vi "Write_LS_Data.vi"(1 "In":T1={"Time"=[], "LI1CH1"=[], "LI1CH2"=[], "LI2CH1"=[], "LI2CH2"=[], "LI3CH1"=[], "LI3CH2"=[], "Field"=[], "N_Level"=[], "H_Level"=[], "Heat_370"=[], "Sorb_Heat"=[], "Still_Heat"=[], "Capacity"=[], "Loss"=[], "Magnet_Temperature"=[], "Lam_Pressure"=[], "Lam_NValve"=[], "370-T1"=[], "370-T2"=[], "370-T3"=[], "370-T4"=[], "370-T5"=[], "370-R1"=[], "370-R2"=[], "370-R3"=[], "370-R4"=[], "370-R5"=[], "372-T1"=[], "372-T2"=[], "372-T3"=[], "372-T4"=[], "372-T5"=[], "372-T6"=[], "372-R1"=[], "372-R2"=[], "372-R3"=[], "372-R4"=[], "372-R5"=[], "372-R6"=[], "Nada"=[nan], "K2440_Res"=[], "K2440_Current"=[], "VTI_Heater"=[], "VTI_NValve"=[], "LS340_Heater"=[], "K6221_Amplitude"=[], "K6221_Frequency"=[], "Cond_Pressure"=[], "Still_Pressure"=[], "FP_Out_Pressure"=[], "Dump_Pressure"=[], "V1"=[], "V2"=[], "V4"=[], "V5"=[], "V9"=[], "Forepump"=[], "Compressor"=[], "K6221_Offset"=[], "BoxTemp"=[], "By"=[], "Bz"=[], "Phi"=[], "heater-recond (%)"=[], "Dewar Pressure "=[], "JT-SP-Control"=[], "350 T1"=[], "350 T2"=[], "350 T3"=[], "350 T4"=[], "350 R1"=[], "350 R2"=[], "350 R3"=[], "350 R4"=[], "Angle"=[], "VTI CH1"=[], "VTI CH2"=[], "VTI CH3"=[], "ColdTrap"=[], "Mischer Pot"=[], "G1 (mbar)"=[], "G3 (mbar) "=[], "G4 (mbar)"=[], "IVC (mbar)"=[], "P2 (mbar) "=[], "Pot mischer (mbar)"=[], "AVS Control Channel (K)"=[], "AVS Control Channel (RES)"=[], "AVS  Channel 5 (RES) "=[], "LI3CH3"=[], "LI3CH4"=[], "LI1CH3"=[], "LI1CH4"=[], "LI2CH3"=[], "LI2CH4"=[], "Volt"=[], "Watt"=[], "Torque Angle"=[], "Dewar heater (W)"=[], "PSU Voltage"=[], "Turbopump"=[], "372-R7"=[], "372-T7"=[], "SIM921 Ch1"=[], " He3 Temp1"=[], " He3 Temp 2"=[], "LI4CH1"=[], "LI4CH2"=[], "372-T8"=[], "372-R8"=[]}) -> (0 "Out":T1={"Time"=[], "LI1CH1"=[], "LI1CH2"=[], "LI2CH1"=[], "LI2CH2"=[], "LI3CH1"=[], "LI3CH2"=[], "Field"=[], "N_Level"=[], "H_Level"=[], "Heat_370"=[], "Sorb_Heat"=[], "Still_Heat"=[], "Capacity"=[], "Loss"=[], "Magnet_Temperature"=[], "Lam_Pressure"=[], "Lam_NValve"=[], "370-T1"=[], "370-T2"=[], "370-T3"=[], "370-T4"=[], "370-T5"=[], "370-R1"=[], "370-R2"=[], "370-R3"=[], "370-R4"=[], "370-R5"=[], "372-T1"=[], "372-T2"=[], "372-T3"=[], "372-T4"=[], "372-T5"=[], "372-T6"=[], "372-R1"=[], "372-R2"=[], "372-R3"=[], "372-R4"=[], "372-R5"=[], "372-R6"=[], "Nada"=[nan], "K2440_Res"=[], "K2440_Current"=[], "VTI_Heater"=[], "VTI_NValve"=[], "LS340_Heater"=[], "K6221_Amplitude"=[], "K6221_Frequency"=[], "Cond_Pressure"=[], "Still_Pressure"=[], "FP_Out_Pressure"=[], "Dump_Pressure"=[], "V1"=[], "V2"=[], "V4"=[], "V5"=[], "V9"=[], "Forepump"=[], "Compressor"=[], "K6221_Offset"=[], "BoxTemp"=[], "By"=[], "Bz"=[], "Phi"=[], "heater-recond (%)"=[], "Dewar Pressure "=[], "JT-SP-Control"=[], "350 T1"=[], "350 T2"=[], "350 T3"=[], "350 T4"=[], "350 R1"=[], "350 R2"=[], "350 R3"=[], "350 R4"=[], "Angle"=[], "VTI CH1"=[], "VTI CH2"=[], "VTI CH3"=[], "ColdTrap"=[], "Mischer Pot"=[], "G1 (mbar)"=[], "G3 (mbar) "=[], "G4 (mbar)"=[], "IVC (mbar)"=[], "P2 (mbar) "=[], "Pot mischer (mbar)"=[], "AVS Control Channel (K)"=[], "AVS Control Channel (RES)"=[], "AVS  Channel 5 (RES) "=[], "LI3CH3"=[], "LI3CH4"=[], "LI1CH3"=[], "LI1CH4"=[], "LI2CH3"=[], "LI2CH4"=[], "Volt"=[], "Watt"=[], "Torque Angle"=[], "Dewar heater (W)"=[], "PSU Voltage"=[], "Turbopump"=[], "372-R7"=[], "372-T7"=[], "SIM921 Ch1"=[], " He3 Temp1"=[], " He3 Temp 2"=[], "LI4CH1"=[], "LI4CH2"=[], "372-T8"=[], "372-R8"=[]})   [LabVIEW 2019]
uses:
  Global/Global Variables/System Monitor Cluster.ctl
  Global/Global Variables/Data_Display_global.vi
  Instrument_Setup.vi
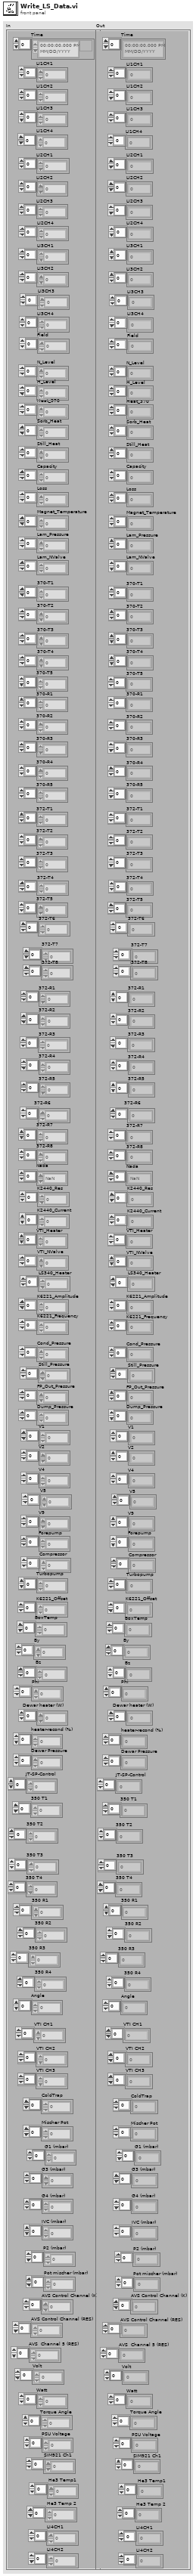
[diagram p1: front panel]
types:
  T1 = typedef "System Monitor Cluster.ctl" = cluster{"Time":timestamp[], "LI1CH1":dbl[], "LI1CH2":dbl[], "LI2CH1":dbl[], "LI2CH2":dbl[], "LI3CH1":dbl[], "LI3CH2":dbl[], "Field":dbl[], "N_Level":dbl[], "H_Level":dbl[], "Heat_370":dbl[], "Sorb_Heat":dbl[], "Still_Heat":dbl[], "Capacity":dbl[], "Loss":dbl[], "Magnet_Temperature":dbl[], "Lam_Pressure":dbl[], "Lam_NValve":dbl[], "370-T1":dbl[], "370-T2":dbl[], "370-T3":dbl[], "370-T4":dbl[], "370-T5":dbl[], "370-R1":dbl[], "370-R2":dbl[], "370-R3":dbl[], "370-R4":dbl[], "370-R5":dbl[], "372-T1":dbl[], "372-T2":dbl[], "372-T3":dbl[], "372-T4":dbl[], "372-T5":dbl[], "372-T6":dbl[], "372-R1":dbl[], "372-R2":dbl[], "372-R3":dbl[], "372-R4":dbl[], "372-R5":dbl[], "372-R6":dbl[], "Nada":dbl[], "K2440_Res":dbl[], "K2440_Current":dbl[], "VTI_Heater":dbl[], "VTI_NValve":dbl[], "LS340_Heater":dbl[], "K6221_Amplitude":dbl[], "K6221_Frequency":dbl[], "Cond_Pressure":dbl[], "Still_Pressure":dbl[], "FP_Out_Pressure":dbl[], "Dump_Pressure":dbl[], "V1":dbl[], "V2":dbl[], "V4":dbl[], "V5":dbl[], "V9":dbl[], "Forepump":dbl[], "Compressor":dbl[], "K6221_Offset":dbl[], "BoxTemp":dbl[], "By":dbl[], "Bz":dbl[], "Phi":dbl[], "heater-recond (%)":dbl[], "Dewar Pressure ":dbl[], "JT-SP-Control":dbl[], "350 T1":dbl[], "350 T2":dbl[], "350 T3":dbl[], "350 T4":dbl[], "350 R1":dbl[], "350 R2":dbl[], "350 R3":dbl[], "350 R4":dbl[], "Angle":dbl[], "VTI CH1":dbl[], "VTI CH2":dbl[], "VTI CH3":dbl[], "ColdTrap":dbl[], "Mischer Pot":dbl[], "G1 (mbar)":dbl[], "G3 (mbar) ":dbl[], "G4 (mbar)":dbl[], "IVC (mbar)":dbl[], "P2 (mbar) ":dbl[], "Pot mischer (mbar)":dbl[], "AVS Control Channel (K)":dbl[], "AVS Control Channel (RES)":dbl[], "AVS  Channel 5 (RES) ":dbl[], "LI3CH3":dbl[], "LI3CH4":dbl[], "LI1CH3":dbl[], "LI1CH4":dbl[], "LI2CH3":dbl[], "LI2CH4":dbl[], "Volt":dbl[], "Watt":dbl[], "Torque Angle":dbl[], "Dewar heater (W)":dbl[], "PSU Voltage":dbl[], "Turbopump":dbl[], "372-R7":dbl[], "372-T7":dbl[], "SIM921 Ch1":dbl[], " He3 Temp1":dbl[], " He3 Temp 2":dbl[], "LI4CH1":dbl[], "LI4CH2":dbl[], "372-T8":dbl[], "372-R8":dbl[]}
  T2 = typedef "LS372-Cluster.ctl" = cluster{"Activate Tsweep":bool, "Setpoint - Manual":dbl, "Rate (K/min)":dbl, "Update Lakeshores":bool, "Still Heater":bool, "Still Power (mW)":dbl, "Manual Heater":bool, "Manual Heater  (mW) ":dbl, "Heater Range":dbl, "P (Gain)":dbl, "I (Reset)":dbl, "D (Rate)":dbl, "Heater Power (mW)":dbl, "MC Thermometer":u16, "MC Temperature":dbl, "LS372-T1":dbl, "LS372 -T2":dbl, "LS372-R1 ":dbl, "LS372-R2":dbl, "LS372-T3":dbl, "LS372-T4":dbl, "LS372-R3 ":dbl, "LS372-R4 \n\n\n\n":dbl, "LS372-T5":dbl, "LS372-T6":dbl, "LS372-R5":dbl, "LS372-R6 ":dbl, "Still Power ist":dbl, "Set Temperatur Sweep main":bool, "Setpoint ist":dbl, "Disable Heater":bool}
  T3 = typedef "LS372_read_only-Cluster.ctl" = cluster{"LS372-T1":dbl, "LS372 -T2":dbl, "LS372-T4":dbl, "LS372-T5":dbl, "LS372-T6":dbl, "LS372-R1 ":dbl, "LS372-R2":dbl, "LS372-R3 ":dbl, "LS372-R4 \n\n\n\n":dbl, "LS372-R5":dbl, "LS372-R6 ":dbl, "LS372-T3":dbl, "Update Lakeshores":bool}
  T4 = typedef "LS370_only_readout_cluster.ctl" = cluster{"LS370 T1":dbl, "LS370 T2":dbl, "LS370 T3":dbl, "LS370 T4":dbl, "LS370 T5":dbl, "LS370 R1":dbl, "LS370 R2":dbl, "LS370 R3":dbl, "LS370 R4":dbl, "LS370 R5":dbl, "LS370 T6":dbl, "LS370 T7":dbl, "LS370 T8":dbl, "LS370 T9":dbl, "LS370 R6":dbl, "LS370 R7":dbl, "LS370 R8":dbl, "LS370 R9":dbl, "LS370 TC-T":dbl, "LS370 TC-R":dbl, "Update Lakeshores":bool}
  T5 = typedef "LS370_Status.ctl" = cluster{"Setpoint":dbl, "MC Heater Output":dbl, "Still Heater Output":dbl, "Sorb  Heater Output":dbl, "LS370 T1":dbl, "LS370 T2":dbl, "LS370 T3":dbl, "LS370 T4":dbl, "LS370 T5":dbl, "LS370 R1":dbl, "LS370 R2":dbl, "LS370 R3":dbl, "LS370 R4":dbl, "LS370 R5":dbl, "LS370 T6":dbl, "LS370 T7":dbl, "LS370 T8":dbl, "LS370 T9":dbl, "LS370 R6":dbl, "LS370 R7":dbl, "LS370 R8":dbl, "LS370 R9":dbl, "LS370 TC-T":dbl, "LS370 TC-R":dbl}
  T6 = typedef "LS350-cluster.ctl" = cluster{"Setpoint":dbl, "Heater Output":dbl, "Setpoint control":dbl, "Enable Setpoint":bool, "LS350 T1":dbl, "LS350 T2":dbl, "LS350 T3":dbl, "LS350 T4":dbl, "LS350 R1":dbl, "LS350 R2":dbl, "LS350 R3":dbl, "LS350 R4":dbl}
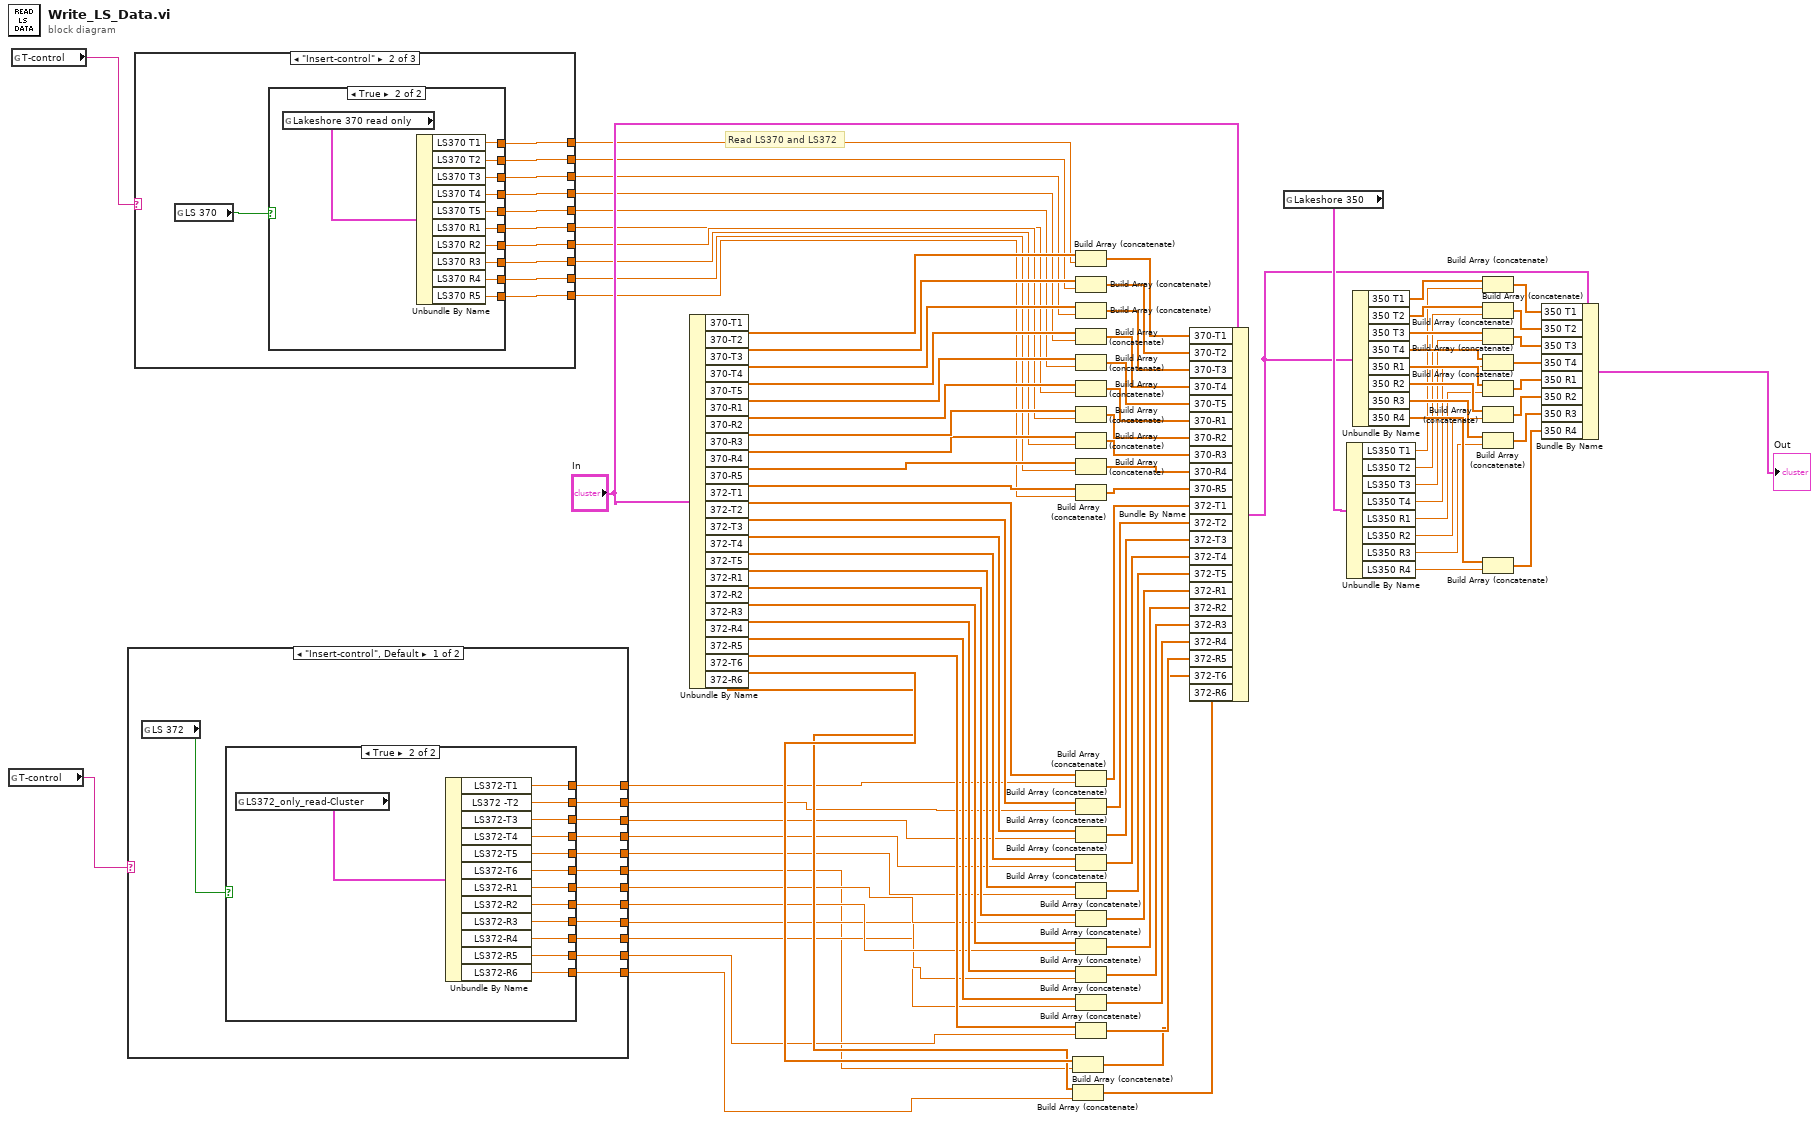
[diagram p0: block diagram]
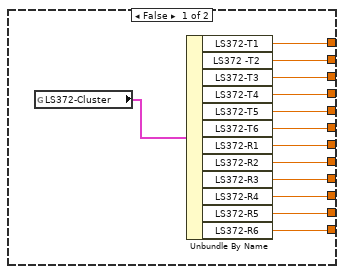
[diagram p2: hidden frame]
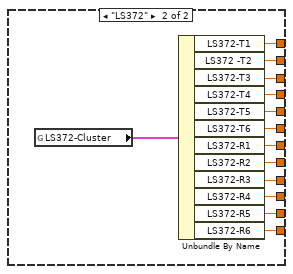
[diagram p3: hidden frame]
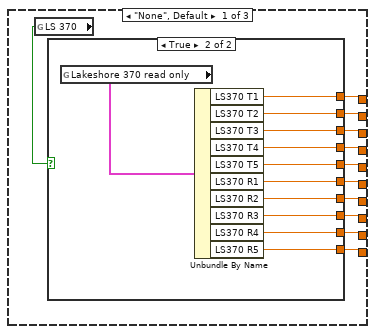
[diagram p4: hidden frame]
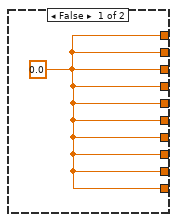
[diagram p5: hidden frame]
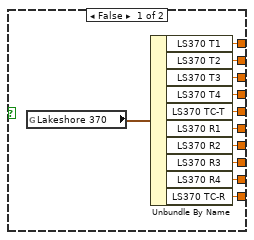
[diagram p6: hidden frame]
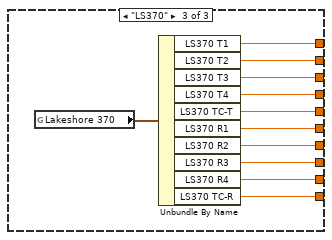
[diagram p7: hidden frame]
diagram:
  # "Read LS370 and LS372"
  n1 = global read "Instrument_Setup.vi" "T-control"() -> (w1:string)
  n2 = global read "Instrument_Setup.vi" "T-control"() -> (w2:string)
  n3 = case shown="\"Insert-control\", Default" w1 {
    tunnel: [w108 w147] -> w14
    tunnel: [w107 w146] -> w13
    tunnel: [w106 w145] -> w12
    tunnel: [w105 w144] -> w11
    tunnel: [w104 w143] -> w10
    tunnel: [w102 w142] -> w9
    tunnel: [w101 w141] -> w8
    tunnel: [w100 w140] -> w7
    tunnel: [w99 w139] -> w6
    tunnel: [w98 w138] -> w5
    tunnel: [w97 w137] -> w4
    tunnel: [w103 w136] -> w3
    frame "Insert-control", Default {
      n4 = global read "Instrument_Setup.vi" "LS 372"() -> (w109:bool)
      n5 = case shown="True" w109 {
        tunnel: [w121 w134] -> w108
        tunnel: [w120 w133] -> w107
        tunnel: [w119 w132] -> w106
        tunnel: [w118 w131] -> w105
        tunnel: [w117 w130] -> w104
        tunnel: [w116 w129] -> w103
        tunnel: [w115 w128] -> w102
        tunnel: [w114 w127] -> w101
        tunnel: [w113 w126] -> w100
        tunnel: [w112 w125] -> w99
        tunnel: [w111 w124] -> w98
        tunnel: [w110 w123] -> w97
        frame False {
          n6 = global read "Data_Display_global.vi" "LS372-Cluster"() -> (w122:T2)
          n7 = Unbundle By Name(w122) -> ("LS372-T1"=w121:dbl, "LS372 -T2"=w120:dbl, "LS372-T3"=w119:dbl, "LS372-T4"=w118:dbl, "LS372-T5"=w117:dbl, "LS372-T6"=w116:dbl, "LS372-R1"=w115:dbl, "LS372-R2"=w114:dbl, "LS372-R3"=w113:dbl, "LS372-R4"=w112:dbl, "LS372-R5"=w111:dbl, "LS372-R6"=w110:dbl)
        }
        frame True {
          n8 = global read "Data_Display_global.vi" "LS372_only_read-Cluster"() -> (w135:T3)
          n9 = Unbundle By Name(w135) -> ("LS372-T1"=w134:dbl, "LS372 -T2"=w133:dbl, "LS372-T3"=w132:dbl, "LS372-T4"=w131:dbl, "LS372-T5"=w130:dbl, "LS372-T6"=w129:dbl, "LS372-R1"=w128:dbl, "LS372-R2"=w127:dbl, "LS372-R3"=w126:dbl, "LS372-R4"=w125:dbl, "LS372-R5"=w124:dbl, "LS372-R6"=w123:dbl)
        }
      }
    }
    frame "LS372" {
      n10 = global read "Data_Display_global.vi" "LS372-Cluster"() -> (w148:T2)
      n11 = Unbundle By Name(w148) -> ("LS372-T1"=w147:dbl, "LS372 -T2"=w146:dbl, "LS372-T3"=w145:dbl, "LS372-T4"=w144:dbl, "LS372-T5"=w143:dbl, "LS372-T6"=w136:dbl, "LS372-R1"=w142:dbl, "LS372-R2"=w141:dbl, "LS372-R3"=w140:dbl, "LS372-R4"=w139:dbl, "LS372-R5"=w138:dbl, "LS372-R6"=w137:dbl)
    }
  }
  n12 = case shown="\"Insert-control\"" w2 {
    tunnel: [w157 w182 w213] -> w55
    tunnel: [w158 w181 w214] -> w54
    tunnel: [w156 w180 w212] -> w53
    tunnel: [w155 w179 w211] -> w52
    tunnel: [w152 w178 w208] -> w51
    tunnel: [w151 w177 w207] -> w50
    tunnel: [w150 w176 w206] -> w49
    tunnel: [w149 w175 w205] -> w48
    tunnel: [w154 w174 w210] -> w47
    tunnel: [w153 w173 w209] -> w46
    frame "None", Default {
      n13 = global read "Instrument_Setup.vi" "LS 370"() -> (w159:bool)
      n14 = case shown="True" w159 {
        tunnel: [w160 w170] -> w158
        tunnel: [w160 w169] -> w157
        tunnel: [w160 w168] -> w156
        tunnel: [w160 w167] -> w155
        tunnel: [w160 w166] -> w154
        tunnel: [w160 w165] -> w153
        tunnel: [w160 w164] -> w152
        tunnel: [w160 w163] -> w151
        tunnel: [w160 w162] -> w150
        tunnel: [w160 w161] -> w149
        frame False {
          w160 = 0.0
        }
        frame True {
          n15 = global read "Data_Display_global.vi" "Lakeshore 370 read only"() -> (w171:T4)
          n16 = Unbundle By Name(w171) -> ("LS370 T1"=w170:dbl, "LS370 T2"=w169:dbl, "LS370 T3"=w168:dbl, "LS370 T4"=w167:dbl, "LS370 T5"=w166:dbl, "LS370 R1"=w165:dbl, "LS370 R2"=w164:dbl, "LS370 R3"=w163:dbl, "LS370 R4"=w162:dbl, "LS370 R5"=w161:dbl)
        }
      }
    }
    frame "Insert-control" {
      n17 = global read "Instrument_Setup.vi" "LS 370"() -> (w172:bool)
      n18 = case shown="True" w172 {
        tunnel: [w192 w202] -> w182
        tunnel: [w191 w203] -> w181
        tunnel: [w190 w201] -> w180
        tunnel: [w189 w200] -> w179
        tunnel: [w188 w197] -> w178
        tunnel: [w187 w196] -> w177
        tunnel: [w186 w195] -> w176
        tunnel: [w185 w194] -> w175
        tunnel: [w184 w199] -> w174
        tunnel: [w183 w198] -> w173
        frame False {
          n19 = global read "Data_Display_global.vi" "Lakeshore 370"() -> (w193:T5)
          n20 = Unbundle By Name(w193) -> ("LS370 T1"=w191:dbl, "LS370 T2"=w192:dbl, "LS370 T3"=w190:dbl, "LS370 T4"=w189:dbl, "LS370 TC-T"=w184:dbl, "LS370 R1"=w183:dbl, "LS370 R2"=w188:dbl, "LS370 R3"=w187:dbl, "LS370 R4"=w186:dbl, "LS370 TC-R"=w185:dbl)
        }
        frame True {
          n21 = global read "Data_Display_global.vi" "Lakeshore 370 read only"() -> (w204:T4)
          n22 = Unbundle By Name(w204) -> ("LS370 T1"=w203:dbl, "LS370 T2"=w202:dbl, "LS370 T3"=w201:dbl, "LS370 T4"=w200:dbl, "LS370 T5"=w199:dbl, "LS370 R1"=w198:dbl, "LS370 R2"=w197:dbl, "LS370 R3"=w196:dbl, "LS370 R4"=w195:dbl, "LS370 R5"=w194:dbl)
        }
      }
    }
    frame "LS370" {
      n23 = global read "Data_Display_global.vi" "Lakeshore 370"() -> (w215:T5)
      n24 = Unbundle By Name(w215) -> ("LS370 T1"=w214:dbl, "LS370 T2"=w213:dbl, "LS370 T3"=w212:dbl, "LS370 T4"=w211:dbl, "LS370 TC-T"=w210:dbl, "LS370 R1"=w209:dbl, "LS370 R2"=w208:dbl, "LS370 R3"=w207:dbl, "LS370 R4"=w206:dbl, "LS370 TC-R"=w205:dbl)
    }
  }
  n25 = Unbundle By Name("In") -> ("370-T1"=w96:dbl[], "370-T2"=w95:dbl[], "370-T3"=w94:dbl[], "370-T4"=w93:dbl[], "370-T5"=w92:dbl[], "370-R1"=w91:dbl[], "370-R2"=w90:dbl[], "370-R3"=w89:dbl[], "370-R4"=w88:dbl[], "370-R5"=w87:dbl[], "372-T1"=w86:dbl[], "372-T2"=w85:dbl[], "372-T3"=w84:dbl[], "372-T4"=w83:dbl[], "372-T5"=w82:dbl[], "372-R1"=w81:dbl[], "372-R2"=w80:dbl[], "372-R3"=w79:dbl[], "372-R4"=w78:dbl[], "372-R5"=w77:dbl[], "372-T6"=w45:dbl[], "372-R6"=w44:dbl[])
  n26 = Build Array (concatenate)(w45, w3) -> (w43:dbl[])
  n27 = Build Array (concatenate)(w44, w4) -> (w42:dbl[])
  n28 = Build Array (concatenate)(w96, w54) -> (w76:dbl[])
  n29 = Build Array (concatenate)(w95, w55) -> (w75:dbl[])
  n30 = Build Array (concatenate)(w94, w53) -> (w74:dbl[])
  n31 = Build Array (concatenate)(w93, w52) -> (w73:dbl[])
  n32 = Build Array (concatenate)(w92, w47) -> (w72:dbl[])
  n33 = Build Array (concatenate)(w91, w46) -> (w71:dbl[])
  n34 = Build Array (concatenate)(w90, w51) -> (w70:dbl[])
  n35 = Build Array (concatenate)(w89, w50) -> (w69:dbl[])
  n36 = Build Array (concatenate)(w88, w49) -> (w68:dbl[])
  n37 = Build Array (concatenate)(w87, w48) -> (w67:dbl[])
  n38 = Build Array (concatenate)(w86, w14) -> (w66:dbl[])
  n39 = Build Array (concatenate)(w85, w13) -> (w65:dbl[])
  n40 = Build Array (concatenate)(w84, w12) -> (w64:dbl[])
  n41 = Build Array (concatenate)(w83, w11) -> (w63:dbl[])
  n42 = Build Array (concatenate)(w82, w10) -> (w62:dbl[])
  n43 = Build Array (concatenate)(w81, w9) -> (w61:dbl[])
  n44 = Build Array (concatenate)(w80, w8) -> (w60:dbl[])
  n45 = Build Array (concatenate)(w79, w7) -> (w56:dbl[])
  n46 = Build Array (concatenate)(w78, w6) -> (w59:dbl[])
  n47 = Build Array (concatenate)(w77, w5) -> (w58:dbl[])
  n48 = Bundle By Name(cluster="In", "370-T1"=w76, "370-T2"=w75, "370-T3"=w74, "370-T4"=w73, "370-T5"=w72, "370-R1"=w71, "370-R2"=w70, "370-R3"=w69, "370-R4"=w68, "370-R5"=w67, "372-T1"=w66, "372-T2"=w65, "372-T3"=w64, "372-T4"=w63, "372-T5"=w62, "372-R1"=w61, "372-R2"=w60, "372-R3"=w56, "372-R4"=w59, "372-R5"=w58, "372-T6"=w43, "372-R6"=w42) -> (w24:T1)
  n49 = global read "Data_Display_global.vi" "Lakeshore 350"() -> (w41:T6)
  n50 = Unbundle By Name(w41) -> ("LS350 T1"=w25:dbl, "LS350 T2"=w26:dbl, "LS350 T3"=w27:dbl, "LS350 T4"=w28:dbl, "LS350 R1"=w29:dbl, "LS350 R2"=w30:dbl, "LS350 R3"=w31:dbl, "LS350 R4"=w32:dbl)
  n51 = Unbundle By Name(w24) -> ("350 T1"=w40:dbl[], "350 T2"=w39:dbl[], "350 T3"=w38:dbl[], "350 T4"=w37:dbl[], "350 R1"=w36:dbl[], "350 R2"=w35:dbl[], "350 R3"=w34:dbl[], "350 R4"=w33:dbl[])
  n52 = Build Array (concatenate)(w40, w25) -> (w22:dbl[])
  n53 = Build Array (concatenate)(w39, w26) -> (w21:dbl[])
  n54 = Build Array (concatenate)(w38, w27) -> (w20:dbl[])
  n55 = Build Array (concatenate)(w37, w28) -> (w19:dbl[])
  n56 = Build Array (concatenate)(w36, w29) -> (w18:dbl[])
  n57 = Build Array (concatenate)(w35, w30) -> (w17:dbl[])
  n58 = Build Array (concatenate)(w34, w31) -> (w16:dbl[])
  n59 = Build Array (concatenate)(w33, w32) -> (w15:dbl[])
  n60 = Bundle By Name(cluster=w24, "350 T1"=w22, "350 T2"=w21, "350 T3"=w20, "350 T4"=w19, "350 R1"=w18, "350 R2"=w17, "350 R3"=w16, "350 R4"=w15) -> (→"Out":T1)
